vi "EOL CAN_Send_Two_Part_Message (2).vi"(0 "Write Session in":refnum<k21>, 1 "Rx Arbitration Id":u32=402522244 format="%.0x", 5 "Read Session in":refnum<k21>, 7 "Tx CAN frame 1":T1={"timestamp"=timestamp(0 s since 1904-01-01), "payload"=[2, 39, 3, 85, 85, 85, 85, 85], "identifier"=402391172, "type"=0, "extended?"=TRUE, "echo?"=FALSE} {"payload" format="%x"; "timestamp" format="%<%.7X\n%x>T"; "type" items=["CAN Data"=0, "CAN Remote"=1, "CAN Bus Error"=2, "CAN 2.0 Data"=8, "CAN FD Data"=16, "CAN FD+BRS Data"=24, "J1939 Data"=192, "Delay"=224, "Log Trigger"=225, "Start Trigger"=226]; "identifier" format="%x"}, 9 "Tx CAN frame 2":T1={"timestamp"=timestamp(0 s since 1904-01-01), "payload"=[2, 39, 3, 85, 85, 85, 85, 85], "identifier"=402391172, "type"=0, "extended?"=TRUE, "echo?"=FALSE} {"payload" format="%x"; "timestamp" format="%<%.7X\n%x>T"; "type" items=["CAN Data"=0, "CAN Remote"=1, "CAN Bus Error"=2, "CAN 2.0 Data"=8, "CAN FD Data"=16, "CAN FD+BRS Data"=24, "J1939 Data"=192, "Delay"=224, "Log Trigger"=225, "Start Trigger"=226]; "identifier" format="%x"}, 11 "error in (no error)":errorcluster, 12 "Retries":i32=3, 13 "Msg Wait Time":u32=100) -> (4 "Response Good?":bool, 6 "Rx Data":u8[](array[numeric]), 10 "TxRx Data":string[][](array[string]), 15 "error out":errorcluster)   [LabVIEW 2018]
uses:
  <vilib>/xnet/xnet.llb/XNET Frame CAN.ctl
  <vilib>/xnet/xnet.llb/XNET Frame Type CAN.ctl
  <vilib>/xnet/xnet.llb/XNET Write (Frame CAN).vi
  <vilib>/xnet/xnet.llb/XNET Read (Frame CAN).vi
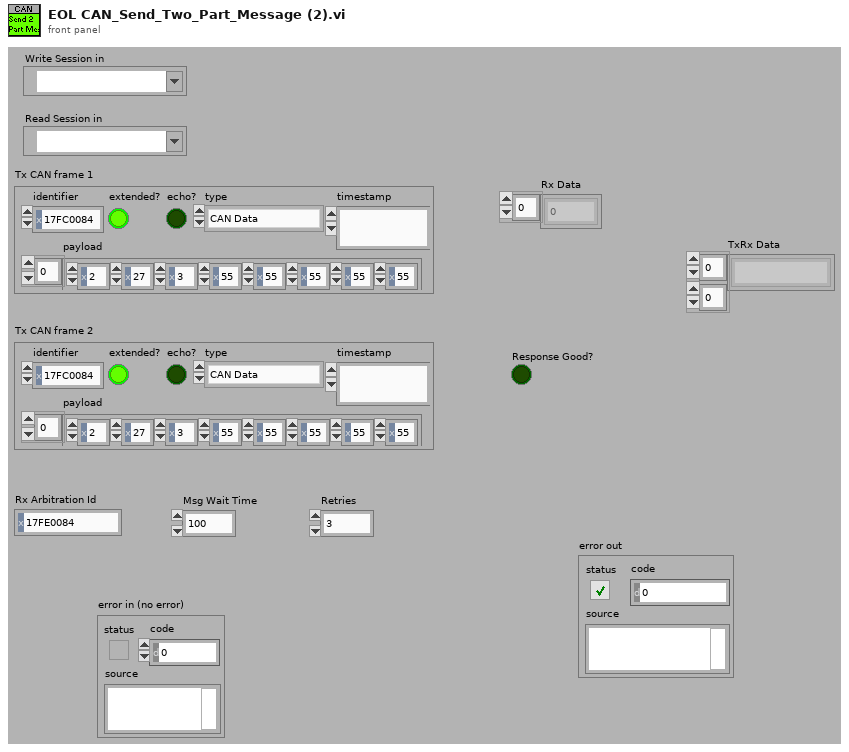
[diagram p1: front panel]
types:
  T1 = typedef "XNET Frame CAN.ctl" = cluster{"timestamp":timestamp, "payload":u8[], "identifier":u32, "type":T2, "extended?":bool, "echo?":bool}
  T2 = typedef "XNET Frame Type CAN.ctl" = u8
  T3 = cluster{"Write Session in":refnum<k21>, "Read Session in":refnum<k21>, "Tx CAN frame 1":T1, "Tx CAN frame 2":T1, "Rx Arbitration Id":u32, "Retry Counter":i32, "Rx Data":u8[], "Response Good?":bool, "TxRx Data":string[][], "Rx Bytes Length":u8, "error in (no error)":errorcluster}
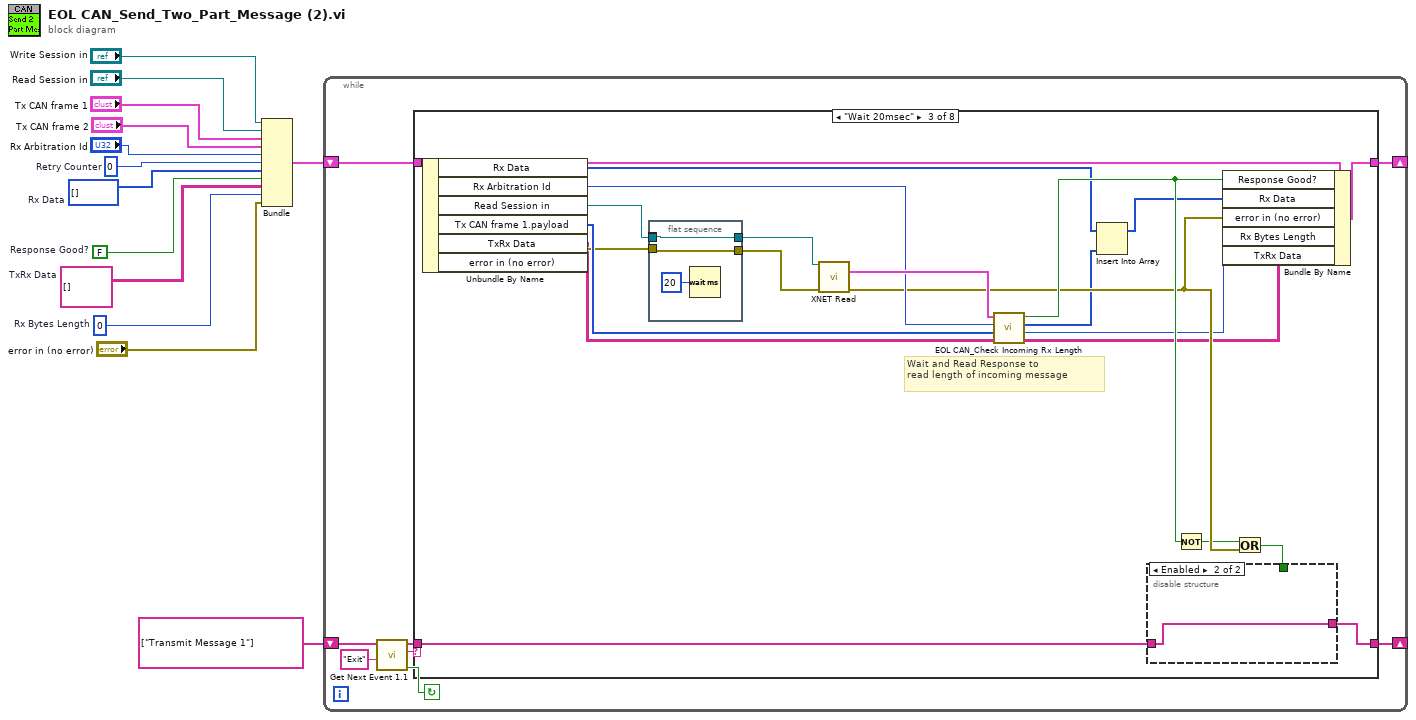
[diagram p0: block diagram]
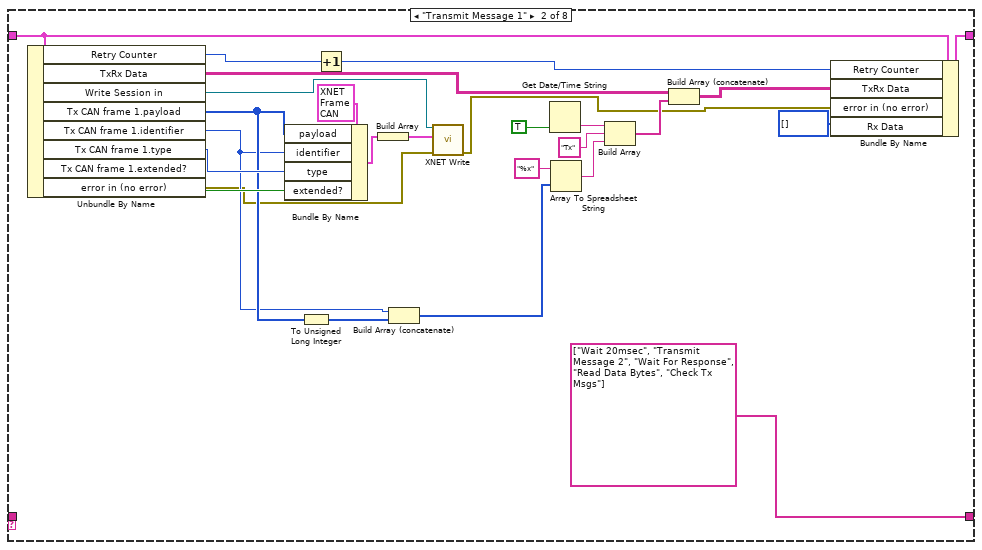
[diagram p3: hidden frame]
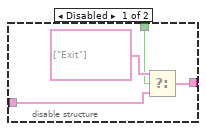
[diagram p4: hidden frame]
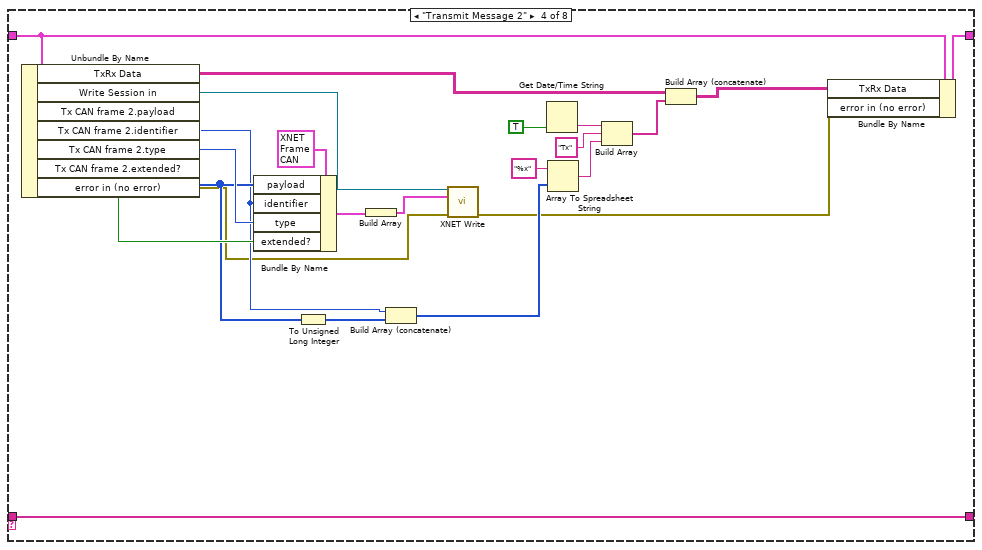
[diagram p5: hidden frame]
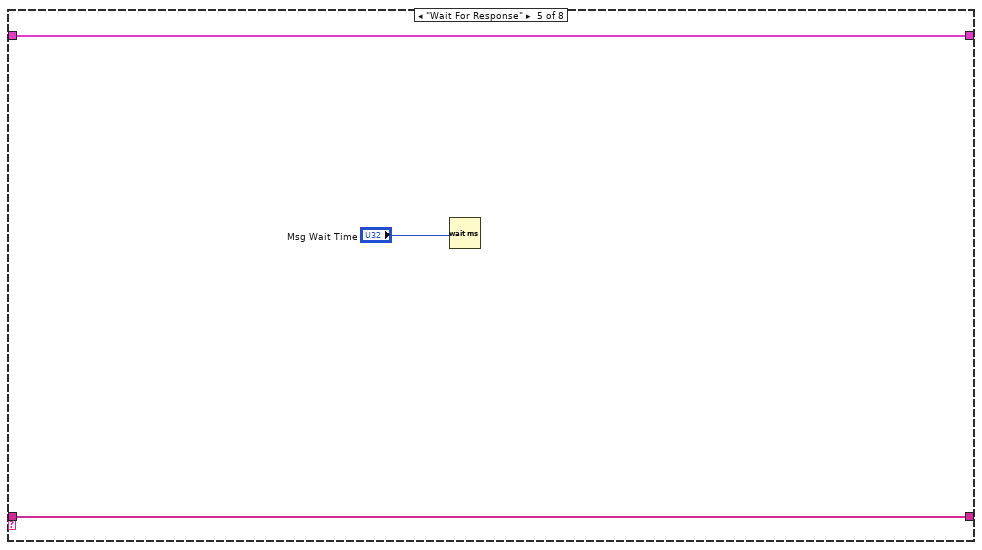
[diagram p6: hidden frame]
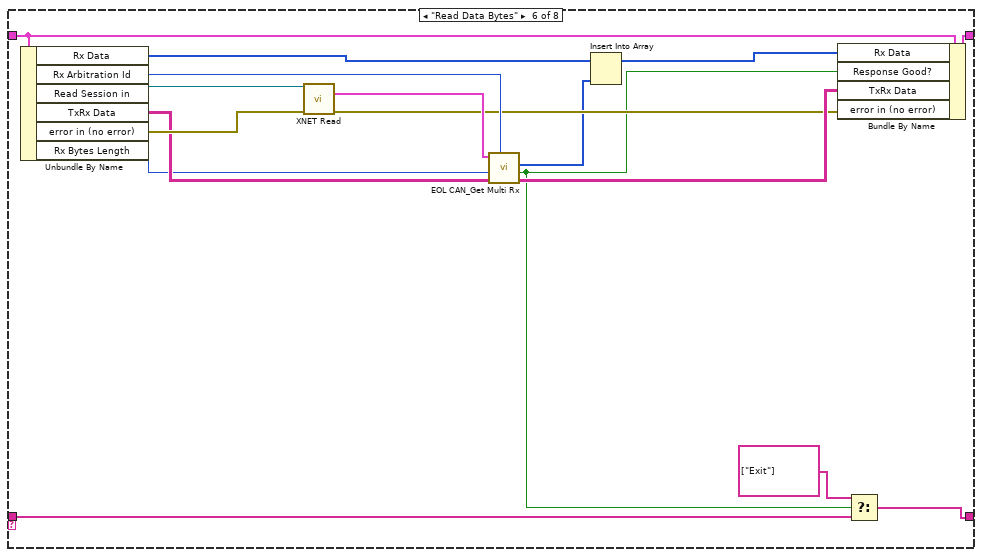
[diagram p7: hidden frame]
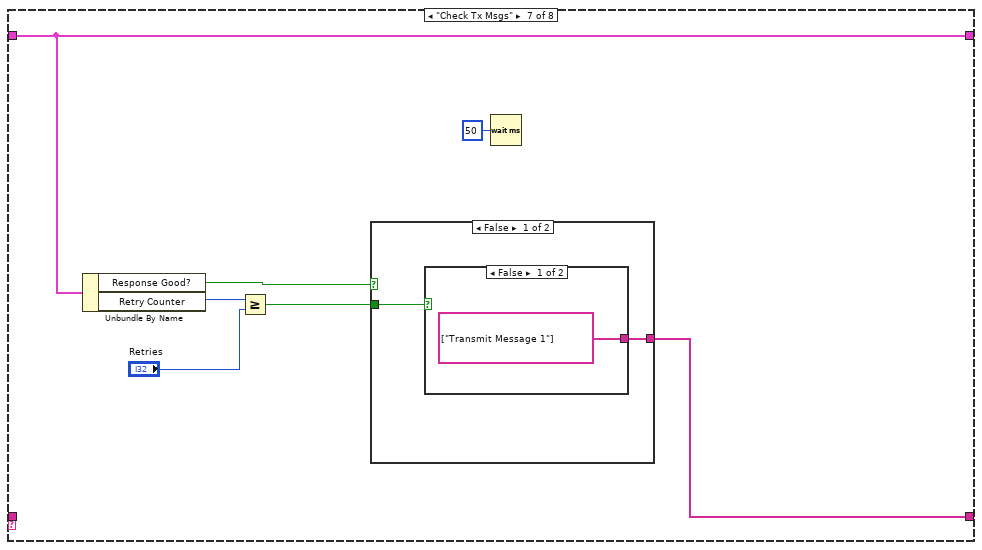
[diagram p8: hidden frame]
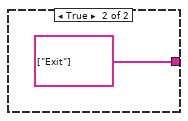
[diagram p9: hidden frame]
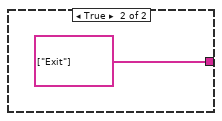
[diagram p10: hidden frame]
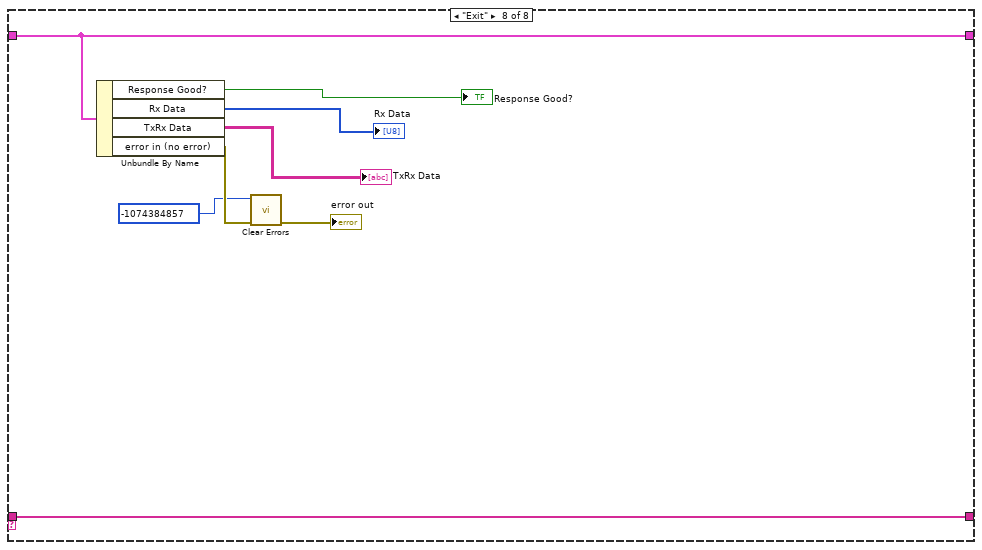
[diagram p11: hidden frame]
diagram:
  w1 = u8[] []  # Rx Data
  w2 = u8 0  # Rx Bytes Length
  w9 = string[][] []  # TxRx Data
  w10 = FALSE  # Response Good?
  w12 = 0  # Retry Counter
  n1 = Bundle("Write Session in"="Write Session in", "Read Session in"="Read Session in", "Tx CAN frame 1"="Tx CAN frame 1", "Tx CAN frame 2"="Tx CAN frame 2", "Rx Arbitration Id"="Rx Arbitration Id", "Retry Counter"=w12, "Rx Data"=w1, "Response Good?"=w10, "TxRx Data"=w9, "Rx Bytes Length"=w2, "error in (no error)"="error in (no error)") -> (w11:T3)  [unwired: 1 in]
  n2 = while {
    shift-right: [w18] -> _
    shift-left: string[] ["Transmit Message 1"] ("event queue out") -> [w17]
    shift-right: [w15] -> _
    shift-left: w11 -> [w16]
    stop <- w21 continue-if-true
    n3 = call <userlib>:"Get Next Event 1.1.vi"("Exit Event"="Exit", "event queue in"=w17) -> ("Condition (Exit:F)"=w21:bool, "next event"=w20:string, "event queue out"=w19:string[])  [unwired: 6 in, 1 out]
    n4 = case shown="\"Wait 20msec\"" w20 {
      tunnel: w19 -> [w23 _ w63 w101 w103 w111 _ w141]
      tunnel: [w23 string[] ["Wait 20msec", "Transmit Message 2", "Wait For Response", "Read Data Bytes", "Check Tx Msgs"] ("event queue out") w62 w101 w103 w110 w126 w141] -> w18
      tunnel: w16 -> [w22 w47 w65 w90 w104 w121 w124 w140]
      tunnel: [w22 w45 w64 w89 w104 w120 w124 w140] -> w15
      frame "Error", Default {
      }
      frame "Transmit Message 1" {
        n5 = Unbundle By Name(w47) -> ("Retry Counter"=w48:i32, "TxRx Data"=w36:string[][], "Write Session in"=w25:refnum<k21>, "Tx CAN frame 1.payload"=w29:u8[], "Tx CAN frame 1.identifier"=w28:u32, "Tx CAN frame 1.type"=w31:T2, "Tx CAN frame 1.extended?"=w30:bool, "error in (no error)"=w27:errorcluster)
        n6 = Bundle By Name(cluster=T1 {"timestamp"=timestamp(0 s since 1904-01-01), "payload"=[], "identifier"=0, "type"=0, "extended?"=FALSE, "echo?"=FALSE} ("CAN frame"), "payload"=w29, "identifier"=w28, "type"=w31, "extended?"=w30) -> (w32:T1)
        n7 = To Unsigned Long Integer(number=w29) -> (unsigned 32bit integer=w44:u32[])
        n8 = Increment(x=w48) -> (x+1=w46:i32)
        n9 = Build Array(w32) -> (w33:T1[])
        n10 = Build Array (concatenate)(w28, w44) -> (w37:u32[])
        n11 = call-poly <vilib>:"XNET Write.vi"("session in"=w25, "data"=w33, "error in (no error)"=w27) -> ("error out"=w26:errorcluster)  [unwired: 11 in, 1 out]
        n12 = Get Date/Time String(want seconds? (F)=TRUE) -> (time string=w40:string)  [unwired: 2 in, 1 out]
        n13 = Array To Spreadsheet String(array=w37, 3:"%x" ("format string")) -> (spreadsheet string=w42:string)  [unwired: 1 in]
        n14 = Build Array(w40, "Tx" ("format string"), w42) -> (w43:string[])
        n15 = Build Array (concatenate)(w36, w43) -> (w35:string[][])
        n16 = Bundle By Name(cluster=w47, "Retry Counter"=w46, "TxRx Data"=w35, "error in (no error)"=w26, "Rx Data"=u8[] []) -> (w45:T3)
      }
      frame "Wait 20msec" {
        # "Wait and Read Response to\nread length of incoming message"
        n17 = Unbundle By Name(w65) -> ("Rx Data"=w54:u8[], "Rx Arbitration Id"=w68:u32, "Read Session in"=w51:refnum<k21>, "Tx CAN frame 1.payload"=w70:u8[], "TxRx Data"=w57:string[][], "error in (no error)"=w61:errorcluster)
        n18 = flat-sequence {
          tunnel: w61 -> [w77]
          tunnel: [w77] -> w60
          tunnel: [w76] -> _
          tunnel: w51 -> [w76]
          tunnel: [w76] -> w50
          frame #0 {
            n19 = Wait (ms)(milliseconds to wait=u32 20) -> ()  [unwired: 1 out]
          }
        }
        n20 = call-poly <vilib>:"XNET Read.vi"("session in"=w50, "error in (no error)"=w60) -> ("data"=w69:T1[], "error out"=w59:errorcluster)  [unwired: 10 in, 2 out]
        n21 = call <userlib>:"EOL CAN_Check Incoming Rx Length.vi"("TxRx Data in"=w57, "Tx"=w70, "Rx Arbitration Id"=w68, "data"=w69) -> ("TxRx Data out"=w55:string[][], "Rx Bytes"=w56:u8, "Rx Data"=w53:u8[], "Response Good?"=w67:bool)  [unwired: 4 in]
        n22 = Insert Into Array(array=w54, new element=w53) -> (w52:u8[])  [unwired: 1 in]
        n23 = Not(x=w67) -> (.not. x?=w58:bool)
        n24 = Bundle By Name(cluster=w65, "Response Good?"=w67, "Rx Data"=w52, "error in (no error)"=w59, "Rx Bytes Length"=w56, "TxRx Data"=w55) -> (w64:T3)
        n25 = Or(x=w58, y=w59) -> (x .or. y?=w66:bool)
        n26 = disable-structure shown="Enabled" {
          disable-tunnel: w66 -> [w73 _]
          disable-tunnel: w63 -> [w72 w75]
          disable-tunnel: [w71 w75] -> w62
          frame Disabled {
            n27 = Select(t=string[] ["Exit"], s=w73, f=w72) -> (s? t:f=w71:string[])
          }
          frame Enabled {
          }
        }
      }
      frame "Transmit Message 2" {
        n28 = Unbundle By Name(w90) -> ("TxRx Data"=w92:string[][], "Write Session in"=w88:refnum<k21>, "Tx CAN frame 2.payload"=w83:u8[], "Tx CAN frame 2.identifier"=w82:u32, "Tx CAN frame 2.type"=w85:T2, "Tx CAN frame 2.extended?"=w84:bool, "error in (no error)"=w80:errorcluster)
        n29 = Bundle By Name(cluster=T1 {"timestamp"=timestamp(0 s since 1904-01-01), "payload"=[], "identifier"=0, "type"=0, "extended?"=FALSE, "echo?"=FALSE} ("CAN frame"), "payload"=w83, "identifier"=w82, "type"=w85, "extended?"=w84) -> (w87:T1)
        n30 = To Unsigned Long Integer(number=w83) -> (unsigned 32bit integer=w100:u32[])
        n31 = Build Array(w87) -> (w81:T1[])
        n32 = Build Array (concatenate)(w82, w100) -> (w93:u32[])
        n33 = call-poly <vilib>:"XNET Write.vi"("session in"=w88, "data"=w81, "error in (no error)"=w80) -> ("error out"=w79:errorcluster)  [unwired: 11 in, 1 out]
        n34 = Get Date/Time String(want seconds? (F)=TRUE) -> (time string=w96:string)  [unwired: 2 in, 1 out]
        n35 = Array To Spreadsheet String(array=w93, 3:"%x" ("format string")) -> (spreadsheet string=w98:string)  [unwired: 1 in]
        n36 = Build Array(w96, "Tx" ("format string"), w98) -> (w99:string[])
        n37 = Build Array (concatenate)(w92, w99) -> (w91:string[][])
        n38 = Bundle By Name(cluster=w90, "TxRx Data"=w91, "error in (no error)"=w79) -> (w89:T3)
      }
      frame "Wait For Response" {
        n39 = Wait (ms)(milliseconds to wait="Msg Wait Time") -> ()  [unwired: 1 out]
      }
      frame "Read Data Bytes" {
        n40 = Unbundle By Name(w121) -> ("Rx Data"=w108:u8[], "Rx Arbitration Id"=w116:u32, "Read Session in"=w119:refnum<k21>, "TxRx Data"=w114:string[][], "error in (no error)"=w117:errorcluster, "Rx Bytes Length"=w113:u8)
        n41 = call-poly <vilib>:"XNET Read.vi"("session in"=w119, "error in (no error)"=w117) -> ("data"=w118:T1[], "error out"=w109:errorcluster)  [unwired: 10 in, 2 out]
        n42 = call <userlib>:"EOL CAN_Get Multi Rx.vi"("Rx Arbitration Id"=w116, "TxRx Data in"=w114, "Rx Bytes Length"=w113, "data"=w118) -> ("TxRx Data out"=w115:string[][], "Response Good?"=w105:bool, "Rx Data"=w107:u8[])  [unwired: 5 in]
        n43 = Insert Into Array(array=w108, new element=w107) -> (w106:u8[])  [unwired: 1 in]
        n44 = Bundle By Name(cluster=w121, "Rx Data"=w106, "Response Good?"=w105, "TxRx Data"=w115, "error in (no error)"=w109) -> (w120:T3)
        n45 = Select(t=string[] ["Exit"], s=w105, f=w111) -> (s? t:f=w110:string[])
      }
      frame "Check Tx Msgs" {
        n46 = Unbundle By Name(w124) -> ("Response Good?"=w127:bool, "Retry Counter"=w128:i32)
        n47 = Greater Or Equal?(x=w128, y="Retries") -> (x >= y?=w125:bool)
        n48 = case shown="False" w127 {
          tunnel: [w129 string[] ["Exit"] ("event queue out")] -> w126
          tunnel: w125 -> [w130 _]
          frame False {
            n49 = case shown="False" w130 {
              tunnel: [string[] ["Transmit Message 1"] ("f") string[] ["Exit"] ("event queue out")] -> w129
              frame False {
              }
              frame True {
              }
            }
          }
          frame True {
          }
        }
        n50 = Wait (ms)(milliseconds to wait=u32 50) -> ()  [unwired: 1 out]
      }
      frame "Exit" {
        n51 = Unbundle By Name(w140) -> ("Response Good?"=→"Response Good?":bool, "Rx Data"=→"Rx Data":u8[], "TxRx Data"=→"TxRx Data":string[][], "error in (no error)"=w137:errorcluster)
        n52 = call <vilib>:"Clear Errors.vi"("error in (no error)"=w137, "specific error code to clear (0: all)"=-1074384857) -> ("error out"=→"error out":errorcluster)  [unwired: 4 in, 1 out]
      }
    }
  }
